vi "运维调试_其他.vi"   [LabVIEW 2016, in "其他.lvlib"]
uses:
  PLC/PLC.lvlib
  <vilib>/ptbypt/NI_PtbyPt.lvlib
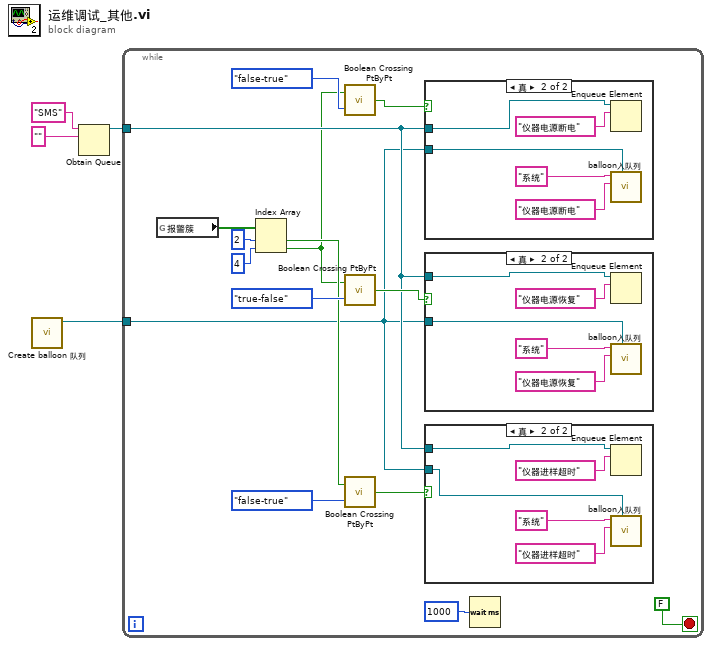
[diagram p0: block diagram]
diagram:
  n1 = call "Create balloon 队列.vi"() -> ("队列输出"=w1:refnum<queue>)  [unwired: 11 in]
  n2 = Obtain Queue(name (unnamed)="SMS" ("名称（未命名）"), element data type="" ("名称（未命名）")) -> (queue out=w2:refnum<queue>)  [unwired: 3 in, 2 out]
  n3 = while {
    tunnel: w2 -> [w13]
    tunnel: w1 -> [w6]
    stop <- FALSE stop-if-true
    n4 = global read "采配水全局变量.vi" "报警簇"() -> (w10:bool[])
    n5 = Index Array(array=w10, index #1=2 ("索引"), index #2=4 ("索引")) -> (element #1=w9:bool, element #2=w7:bool)
    n6 = call <vilib>:"Boolean Crossing PtByPt.vi"("direction"=enum16{"either", "false-true", "true-false"}."false-true", "input"=w7) -> ("crossing"=w16:bool)  [unwired: 1 in]
    n7 = call <vilib>:"Boolean Crossing PtByPt.vi"("direction"=enum16{"either", "false-true", "true-false"}."true-false", "input"=w7) -> ("crossing"=w14:bool)  [unwired: 1 in]
    n8 = call <vilib>:"Boolean Crossing PtByPt.vi"("direction"=enum16{"either", "false-true", "true-false"}."false-true", "input"=w9) -> ("crossing"=w11:bool)  [unwired: 1 in]
    n9 = case shown="真" w16 {
      tunnel: w13 -> [_ w34]
      tunnel: w6 -> [_ w32]
      frame False {
      }
      frame True {
        n10 = Enqueue Element(queue=w34, element="仪器电源断电" ("元素")) -> ()  [unwired: 2 in, 3 out]
        n11 = call "balloon入队列.vi"("队列"=w32, "故障信息"="仪器电源断电" ("元素"), "参数名称"="系统") -> ()  [unwired: 8 in, 1 out]
      }
    }
    n12 = case shown="真" w14 {
      tunnel: w13 -> [_ w27]
      tunnel: w6 -> [_ w26]
      frame False {
      }
      frame True {
        n13 = Enqueue Element(queue=w27, element="仪器电源恢复" ("元素")) -> ()  [unwired: 2 in, 3 out]
        n14 = call "balloon入队列.vi"("队列"=w26, "故障信息"="仪器电源恢复" ("元素"), "参数名称"="系统") -> ()  [unwired: 8 in, 1 out]
      }
    }
    n15 = case shown="真" w11 {
      tunnel: w13 -> [_ w24]
      tunnel: w6 -> [_ w22]
      frame False {
      }
      frame True {
        n16 = Enqueue Element(queue=w24, element="仪器进样超时" ("元素")) -> ()  [unwired: 2 in, 3 out]
        n17 = call "balloon入队列.vi"("队列"=w22, "故障信息"="仪器进样超时" ("元素"), "参数名称"="系统") -> ()  [unwired: 8 in, 1 out]
      }
    }
    n18 = Wait (ms)(milliseconds to wait=u32 1000 ("等待时间（毫秒）")) -> ()  [unwired: 1 out]
  }
